vi "Set Picture Control Scaling to Fit.vi"(7 "Erase First? (Default: True)":bool=TRUE, 8 "error in (no error)":errorcluster, 10 "Image Size":T2, 11 "Picture in":refnum<vi>) -> (0 "error out":errorcluster, 3 "Image Draw Offset":T1)   [LabVIEW 2020, in "AR Example.lvlib" / "UI.lvclass"]
uses:
  UI.lvclass
  g_ar_toolkit.image/Image Draw Offset.ctl
  g_ar_toolkit.common/Image Size (Integer).ctl
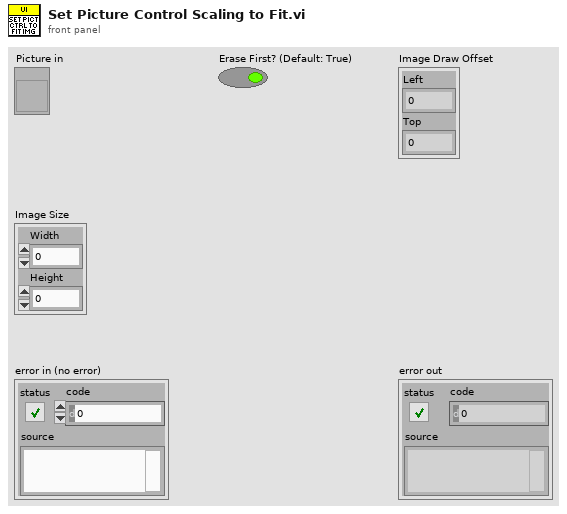
[diagram p1: front panel]
types:
  T1 = typedef "g_ar_toolkit.image.lvlib/Image Draw Offset.ctl" = cluster{"Left":i16, "Top":i16}
  T2 = typedef "g_ar_toolkit.common.lvlib/Image Size (Integer).ctl" = cluster{"Width":u16, "Height":u16}
  T3 = typedef "LVBoundsTypeDef.ctl" = cluster{"Width":u32, "Height":u32}
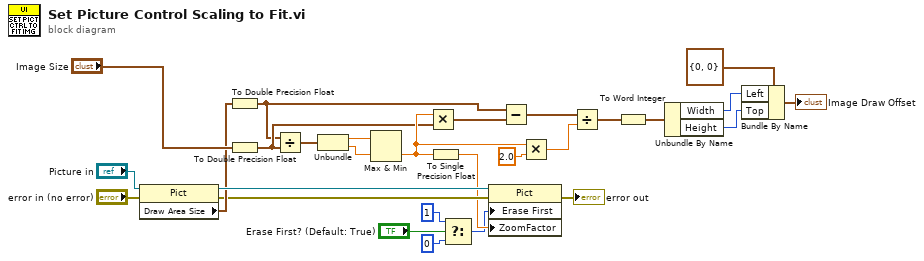
[diagram p0: block diagram]
diagram:
  n1 = property on="Property Node" class="Pict"(reference="Picture in", error in="error in (no error)") -> (reference out=w28:refnum<vi>, error out=w9:errorcluster, "Draw Area Size"=w11:T3)
  n2 = To Double Precision Float(number=w11) -> (double precision float=w13:cluster{"Width":dbl, "Height":dbl})
  n3 = To Double Precision Float(number="Image Size") -> (double precision float=w14:cluster{"Width":dbl, "Height":dbl})
  n4 = Divide(x=w13, y=w14) -> (x/y=w6:cluster{"Width":dbl, "Height":dbl})
  n5 = Unbundle(w6) -> ("Width"=w8:dbl, "Height"=w7:dbl)
  n6 = Max & Min(x=w8, y=w7) -> (min(x,y)=w22:dbl)  [unwired: 1 out]
  n7 = Multiply(x=w22, y=w14) -> (x*y=w10:cluster{"Width":dbl, "Height":dbl})
  n8 = To Single Precision Float(number=w22) -> (single precision float=w5:sgl)
  n9 = Select(t=u8 1 ("Erase First"), s="Erase First? (Default: True)", f=u8 0) -> (s? t:f=w2:u8)
  n10 = property on="Property Node" class="Pict"(reference=w28, error in=w9, "Erase First"=w2, "ZoomFactor"=w5) -> (error out=→"error out":errorcluster)  [unwired: 1 out]
  n11 = Subtract(x=w13, y=w10) -> (x-y=w12:cluster{"Width":dbl, "Height":dbl})
  n12 = Multiply(x=w22, y=2.0) -> (x*y=w21:dbl)
  n13 = Divide(x=w12, y=w21) -> (x/y=w16:cluster{"Width":dbl, "Height":dbl})
  n14 = To Word Integer(number=w16) -> (16bit integer=w18:cluster{"Width":i16, "Height":i16})
  n15 = Unbundle By Name(w18) -> ("Width"=w19:i16, "Height"=w20:i16)
  n16 = Bundle By Name(cluster=T1 {"Left"=0, "Top"=0} ("Image Draw Offset"), "Left"=w19, "Top"=w20) -> (→"Image Draw Offset":T1)
